vi "Get Only Valid Waveform.vi"(8 "Last Valid Point":i32, 10 "Input Waveform Graph":i16[](graph), 11 "First Valid Point":i32) -> (2 "Valid Waveform Graph":i16[](graph))   [LabVIEW 2015, in "LeCroy Wave Series.lvlib"]
doc: "Remove invalide points from curve."
uses:
  <instrlib>/LeCroy Wave Series/LeCroy Wave Series.lvlib
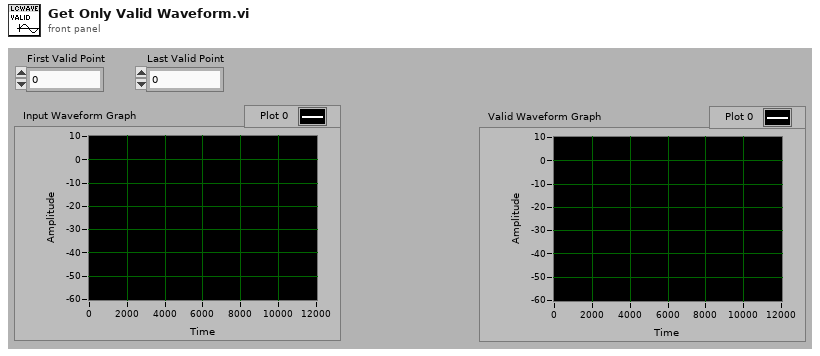
[diagram p1: front panel]
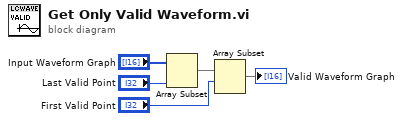
[diagram p0: block diagram]
diagram:
  n1 = Array Subset(array="Input Waveform Graph", length="Last Valid Point") -> (w4:i16[])  [unwired: 1 in]
  n2 = Array Subset(array=w4, index="First Valid Point") -> (→"Valid Waveform Graph":i16[])  [unwired: 1 in]
